vi "Sorensen M9A Series Basic Usage.vi"() -> ()   [LabVIEW 2021]
doc: "This VI is a simple example to show how the Sorensen power supply VIs can be assembled into one VI. Note that not all instrument VIs were included."
uses:
  Sorensen M9A Series.lvlib
panel:
  in  "VISA resource name":refnum<visa-resource-name>
  out "Output Voltage (V)":dbl format="%.2f"
  out "Output Current (A)":dbl format="%.2f"
  in  "Set Current (A)":dbl format="%.2f"
  in  "Set Voltage (V)":dbl format="%.2f"
  in  "Seconds to Wait Between Set and Check (s)":i32=1
  in  "Output (T: ON)":bool=TRUE
  in  "Hold (F: Off)":bool
  # "(c) 2004-2009 National Instruments.  ALL RIGHTS RESERVED."
  # "Sorensen M9A Basic Usage Example"
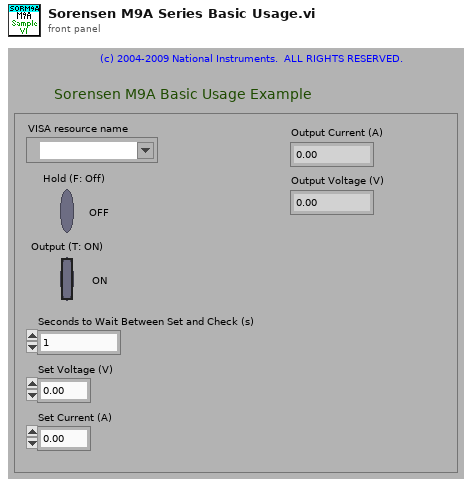
[diagram p1: front panel]
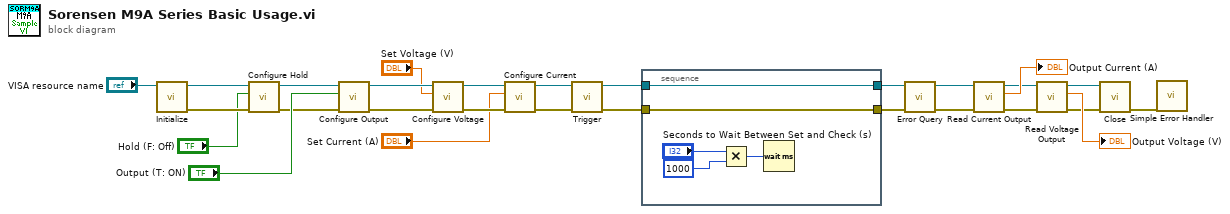
[diagram p0: block diagram]
diagram:
  n1 = call "Initialize.vi"("VISA resource name"="VISA resource name") -> ("error out"=w26:errorcluster, "VISA resource name out"=w27:refnum<visa-resource-name>)  [unwired: 9 in]
  n2 = call "Configure Hold.vi"("error in (no error)"=w26, "Hold (F:OFF)"="Hold (F: Off)", "VISA resource name"=w27) -> ("error out"=w22:errorcluster, "VISA resource name out"=w23:refnum<visa-resource-name>)  [unwired: 7 in]
  n3 = call "Configure Output.vi"("error in (no error)"=w22, "Output (F:OFF)"="Output (T: ON)", "VISA resource name"=w23) -> ("error out"=w20:errorcluster, "VISA resource name out"=w21:refnum<visa-resource-name>)  [unwired: 7 in]
  n4 = call "Configure Voltage.vi"("error in (no error)"=w20, "Set Voltage (0 V)"="Set Voltage (V)", "VISA resource name"=w21) -> ("error out"=w17:errorcluster, "VISA resource name out"=w18:refnum<visa-resource-name>)  [unwired: 7 in]
  n5 = call "Configure Current.vi"("error in (no error)"=w17, "Set Current (0 A)"="Set Current (A)", "VISA resource name"=w18) -> ("error out"=w14:errorcluster, "VISA resource name out"=w15:refnum<visa-resource-name>)  [unwired: 7 in]
  n6 = call "Trigger.vi"("error in (no error)"=w14, "VISA resource name"=w15) -> ("error out"=w12:errorcluster, "VISA resource name out"=w13:refnum<visa-resource-name>)  [unwired: 8 in]
  n7 = stacked-sequence {
    tunnel: w13 -> [w30]
    tunnel: w12 -> [w29]
    tunnel: [w30] -> w11
    tunnel: [w29] -> w10
    frame #0 {
      n8 = Multiply(x="Seconds to Wait Between Set and Check (s)", y=1000) -> (x*y=w32:i32)
      n9 = Wait (ms)(milliseconds to wait=w32) -> ()  [unwired: 1 out]
    }
  }
  n10 = call "Error Query.vi"("error in (no error)"=w10, "VISA resource name"=w11) -> ("error out"=w2:errorcluster, "VISA resource name out"=w3:refnum<visa-resource-name>)  [unwired: 6 in, 2 out]
  n11 = call "Read Current Output.vi"("error in (no error)"=w2, "VISA resource name"=w3) -> ("error out"=w7:errorcluster, "Current Output (A)"=→"Output Current (A)":dbl, "VISA resource name out"=w8:refnum<visa-resource-name>)  [unwired: 7 in]
  n12 = call "Read Voltage Output.vi"("error in (no error)"=w7, "VISA resource name"=w8) -> ("error out"=w4:errorcluster, "Voltage Output (V)"=→"Output Voltage (V)":dbl, "VISA resource name out"=w5:refnum<visa-resource-name>)  [unwired: 7 in]
  n13 = call "Close.vi"("error in (no error)"=w4, "VISA resource name"=w5) -> ("error out"=w1:errorcluster)  [unwired: 9 in]
  n14 = call <vilib>:"Simple Error Handler.vi"("error in (no error)"=w1) -> ()  [unwired: 4 in, 5 out]
